vi "TCP File Receiver.vi"() -> ()   [LabVIEW 2015]
doc: "This VI supports a TCP file transfer application on an sbRIO target. In the TCP File Sender.vi, data is read from an FPGA personality, stored to a spreadsheet file, then transfered via TCP. The TCP File Receiver.vi will then collect the spreadsheet file and format the data for display.\n\nInstructions for Use:\n1. Open and run TCP File Receiver.vi. It will wait up to 60 seconds for a connection on the specified port.\n2. Open and run TCP File Sender.vi\n3. View the results on the waveform graph below."
uses:
  <vilib>/Utility/file.llb/Read Delimited Spreadsheet (DBL).vi
panel:
  in  "File Path":path=path "C:/Additional Exercises/15 - TCP File Transfer/Waveform Data.xml"
  out "Waveform Graph":dbl[][](graph)
  in  "Port":u16=5280
  # "This VI reads a file transfered from the eval kit over TCP. In the TCP File Sender.vi running\non the target, sine wave data is read from the FPGA, stored to a spreadsheet file, then\ntransmitted over the network via TCP. This TCP File Receiver.vi then collects the spreadsheet \nfile and formats the data to display. Specify the file path on your host computer below.\n\nInstructions for Use:\n1. Run TCP File Receiver.vi. It will wait up to 60 seconds for a connection on the specified port.\n2. Open and run TCP File Sender.vi on your evaluation kit.\n3. Wait briefly and view the results on the waveform graph below."
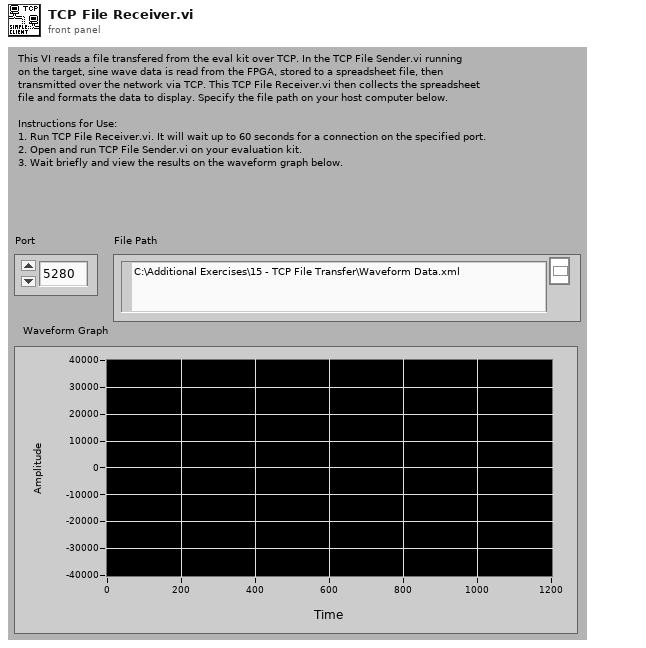
[diagram p1: front panel]
types:
  T1 = enum16{"open", "replace", "create", "open or create", "replace or create", "replace or create with confirmation"}
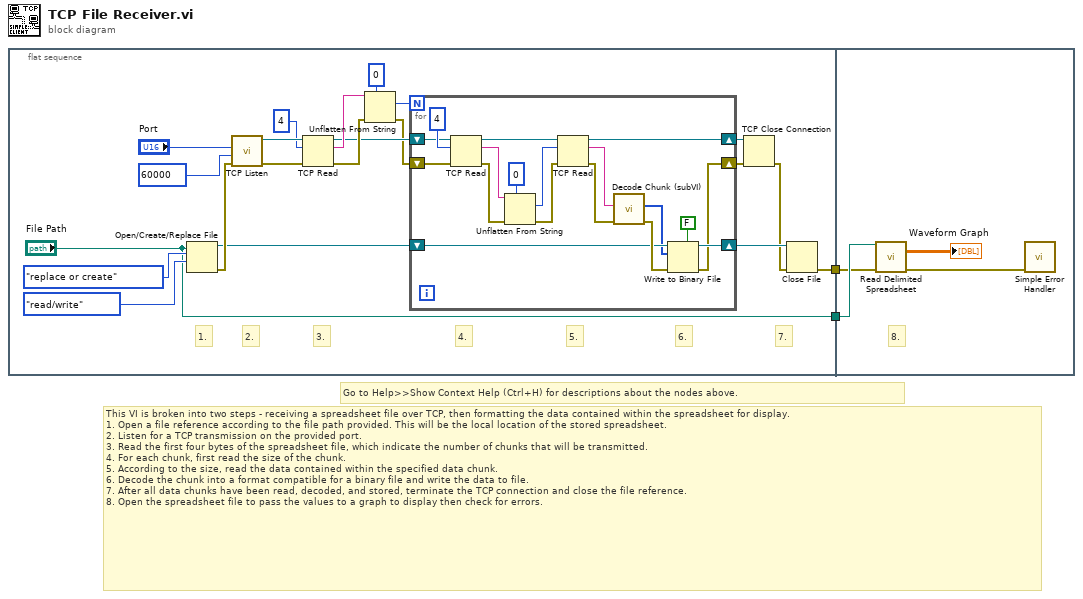
[diagram p0: block diagram]
diagram:
  # "Go to Help>>Show Context Help (Ctrl+H) for descriptions about the nodes above."
  # "This VI is broken into two steps - receiving a spreadsheet file over TCP, then formatting the data contained within the spreadsheet for display.\n1. Open a file reference according to the file path provided. This will be the local location of the stored spreadsheet.\n2. Listen for a TCP transmission on the provided port.\n3. Read the first four bytes of the spreadsheet file, which indicate the number of chunks that will be transmitted.\n4. For each chunk, first read the size of the chunk.\n5. According to the size, read the data contained within the specified data chunk.\n6. Decode the chunk into a format compatible for a binary file and write the data to file.\n7. After all data chunks have been read, decoded, and stored, terminate the TCP connection and close the file reference.\n8. Open the spreadsheet file to pass the values to a graph to display then check for errors."
  n1 = flat-sequence {
    tunnel: ["File Path"] -> w2
    tunnel: [w3] -> w1
    tunnel: w2 -> [w45]
    tunnel: w1 -> [w43]
    frame #0 {
      # "6."
      # "5."
      # "4."
      # "7."
      # "3."
      # "2."
      # "1."
      n2 = Open/Create/Replace File(file path (use dialog)="File Path", operation (0:open)=T1."replace or create", access (0:read/write)=enum16{"read/write", "read-only", "write-only"}."read/write") -> (refnum out=w11:refnum<file>, error out=w21:errorcluster)  [unwired: 1 in, 3 out]
      n3 = call <vilib>:"TCP Listen.vi"("error in (no error)"=w21, "timeout ms (wait forever: -1)"=60000, "port"="Port") -> ("error out"=w18:errorcluster, "connection ID"=w19:refnum<k5>)  [unwired: 1 in, 6 out]
      n4 = TCP Read(connection ID=w19, bytes to read=4, error in (no error)=w18) -> (connection ID out=w12:refnum<k5>, data out=w15:string, error out=w16:errorcluster)  [unwired: 2 out]
      n5 = Unflatten From String(type=0 ("bytes to read"), binary string=w15, error in (no error)=w16) -> (value=w13:i32, error out=w10:errorcluster)  [unwired: 3 out]
      n6 = for {
        N: w13 -> [_]
        shift-right: [w28] -> w7
        shift-left: w12 -> [w39]
        shift-right: [w26] -> w8
        shift-left: w10 -> [w33]
        shift-right: [w29] -> w9
        shift-left: w11 -> [w31]
        n7 = TCP Read(connection ID=w39, bytes to read=4, error in (no error)=w33) -> (connection ID out=w38:refnum<k5>, data out=w25:string, error out=w37:errorcluster)  [unwired: 2 out]
        n8 = Unflatten From String(type=0 ("bytes to read"), binary string=w25, error in (no error)=w37) -> (value=w34:i32, error out=w36:errorcluster)  [unwired: 3 out]
        n9 = TCP Read(connection ID=w38, bytes to read=w34, error in (no error)=w36) -> (connection ID out=w28:refnum<k5>, data out=w35:string, error out=w27:errorcluster)  [unwired: 2 out]
        n10 = call "Decode Chunk (subVI).vi"("error in (no error)"=w27, "Chunk (without size)"=w35) -> ("error out"=w32:errorcluster, "Flattened Data"=w24:u8[])  [unwired: 8 out]
        n11 = Write to Binary File(file (use dialog)=w31, data=w24, error in=w32, 5:FALSE ("prepend array or string size? (T)")) -> (refnum out=w29:refnum<file>, error out=w26:errorcluster)  [unwired: 3 out]
      }
      n12 = TCP Close Connection(connection ID=w7, error in (no error)=w8) -> (error out=w6:errorcluster)  [unwired: 2 out]
      n13 = Close File(refnum=w9, error in=w6) -> (error out=w3:errorcluster)  [unwired: 1 out]
    }
    frame #1 {
      # "8."
      n14 = call-poly <vilib>:"Read Delimited Spreadsheet.vi"("file path (dialog if empty)"=w45, "error in (no error)"=w43) -> ("all rows"=→"Waveform Graph":dbl[][], "error out"=w42:errorcluster)  [unwired: 8 in, 4 out]
      n15 = call <vilib>:"Simple Error Handler.vi"("error in (no error)"=w42) -> ()  [unwired: 4 in, 5 out]
    }
  }
